vi "Stop.vi"(8 "error in (no error)":errorcluster, 11 "Scope PXI Base CFG in":refnum<class "Scope PXI Base CFG.lvclass">) -> (0 "error out":errorcluster, 3 "Scope PXI Base CFG out":refnum<class "Scope PXI Base CFG.lvclass">)   [LabVIEW 2023, in "Scope PXI Base CFG.lvclass"]
uses:
  Scope PXI Base CFG.lvclass
  Scope PXI Base CFG.lvclass/Scope PXI Base CFG.ctl
  <vilib>/Utility/error.llb/Error Cluster From Error Code.vi
  <vilib>/ErrorRing/Error Ring.xnode
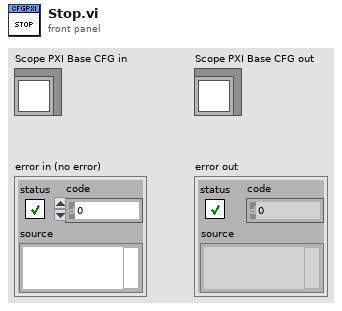
[diagram p1: front panel]
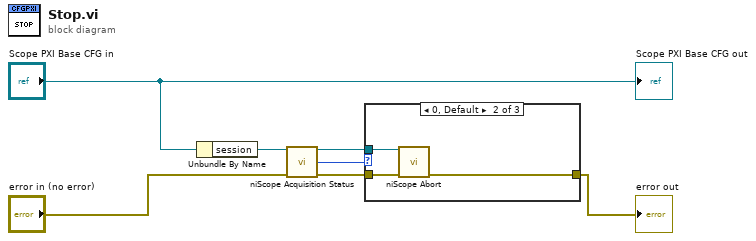
[diagram p0: block diagram]
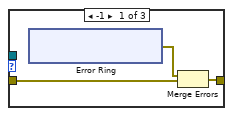
[diagram p2: hidden frame]
diagram:
  n1 = Unbundle By Name("Scope PXI Base CFG in") -> ("session"=w1:refnum<k15>)
  n2 = call <instrlib>:"niScope Acquisition Status.vi"("instrument handle"=w1, "error in"="error in (no error)") -> ("instrument handle out"=w3:refnum<k15>, "acquisition status"=w2:i32, "error out"=w4:errorcluster)  [unwired: 11 in]
  n3 = case shown="0, Default" w2 {
    tunnel: [w10 w18 w19] -> w6
    tunnel: w4 -> [w8 w17 w19]
    tunnel: w3 -> [_ w16 _]
    frame -1 {
      n4 = xnode "Error Ring"() -> ("error out"=w9:errorcluster)
      n5 = Merge Errors(w9, w8) -> (w10:errorcluster)
    }
    frame 0, Default {
      n6 = call <instrlib>:"niScope Abort.vi"("instrument handle"=w16, "error in"=w17) -> ("error out"=w18:errorcluster)  [unwired: 12 in, 1 out]
    }
    frame 1 {
    }
  }
  "error out" <- w6
  "Scope PXI Base CFG out" <- "Scope PXI Base CFG in"
